vi "Force2Voltage_Linearizer_v0.vi"(6 "Z_offset [mm]":fxp<+/-,26,3>=0.02499997615814209, 7 "Scale Factor":fxp<+,10,10>=619.0, 8 "Z [mm]":fxp<+/-,26,3>, 9 "F_B [N]":fxp<+/-,25,3>, 10 "F_G [N]":fxp<+/-,25,3>, 11 "F_R [N]":fxp<+/-,25,3>) -> (1 "V_B [V]":fxp<+/-,20,5>, 2 "V_G [V]":fxp<+/-,20,5>, 3 "V_R [V]":fxp<+/-,20,5>)   [LabVIEW 2020, in "FPGA functions.lvlib"]
doc: "Linearizing actuation force to electrode voltages. \n\nThis implements the feedback linearization block!"
uses:
  FPGA functions.lvlib
  <vilib>/Platform/TimedLoop/XDataNode/timing_clust.ctl
  <vilib>/Platform/TimedLoop/XDataNode/nitl_modes.ctl
  <vilib>/Platform/TimedLoop/XDataNode/wakeup.ctl
  <vilib>/rvi/FXPMathLib/FxpSqrt/subVIs/nifxpmath_Sqrt_SimConfig.ctl
  <vilib>/fxp/LVFixedPointOverflowPolicyTypeDef.ctl
  <vilib>/rvi/Emulation/niFpgaSctlEmulationGetInTimedLoop.vi
  <vilib>/rvi/Emulation/niFpgaEmulationReportErrorSimple.vi
  <vilib>/rvi/Emulation/niFpgaGetClockAttributes.vi
  <vilib>/rvi/Emulation/niFpgaCriticalErrorInLSC.vi
  <vilib>/rvi/FXPMathLib/FxpSqrt/simVIs/DllSqrtTemp_sub.vi
  <vilib>/Platform/TimedLoop/XDataNode/XDataNode.xnode
  <vilib>/rvi/FXPMathLib/FxpSqrt/XNode/nifxpmath_Sqrt.xnode
  <vilib>/rvi/FXPMathLib/FxpAdd/XNode/nifxpmath_Add.xnode
  <vilib>/rvi/FXPMathLib/FxpMul/XNode/nifxpmath_Multiplier.xnode
  <vilib>/Platform/TimedLoop/XDataNode/XDNodeRunTimeDep.lvlib
  <vilib>/rvi/FXPMathLib/sim/FxpSim.dll
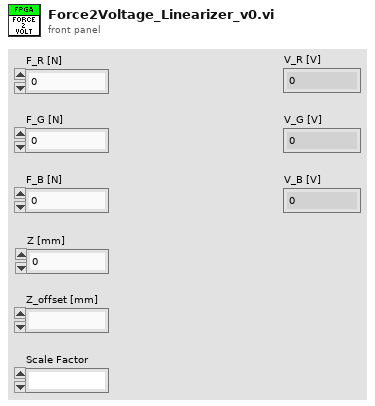
[diagram p1: front panel]
types:
  T1 = typedef "XDNodeRunTimeDep.lvlib/timing_clust.ctl" = cluster{"Expected End [f-1]":u64, "Actual End [f-1]":u64, "Finished Late? [f-1]":bool, "Expected End [i-1]":u64, "Actual End [i-1]":u64, "Finished Late? [i-1]":bool, "Expected Start [i]":u64, "Actual Start [i]":u64, "Expected Start [f]":u64, "Actual Start [f]":u64, "Source Name":string, "Structure Name":string, "Period":i64, "Deadline":i64, "Offset":i64, "Start":i64, "Priority":i32, "Timeout":i32, "Mode":T2, "Wakeup Reason":T3, "Error":errorcluster, "Source Type":string, "Secondary Source Type":string, "Global End Time":u64, "Global Start Time":u64, "Frame Duration":u64, "Iteration Duration":u64, "Assigned CPU":i32, "I/O Scan Engine Mode":u32}
  T2 = typedef "XDNodeRunTimeDep.lvlib/nitl_modes.ctl" = enum32{"No Change", "Process missed periods, maintain original phase", "Discard missed periods, maintain original phase", "Process missed periods, ignore original phase", "Discard missed periods, ignore original phase"}
  T3 = typedef "XDNodeRunTimeDep.lvlib/wakeup.ctl" = enum32{"Normal", "Aborted", "Asynchronous wakeup", "Timing source error", "Timed loop error", "Timeout"}
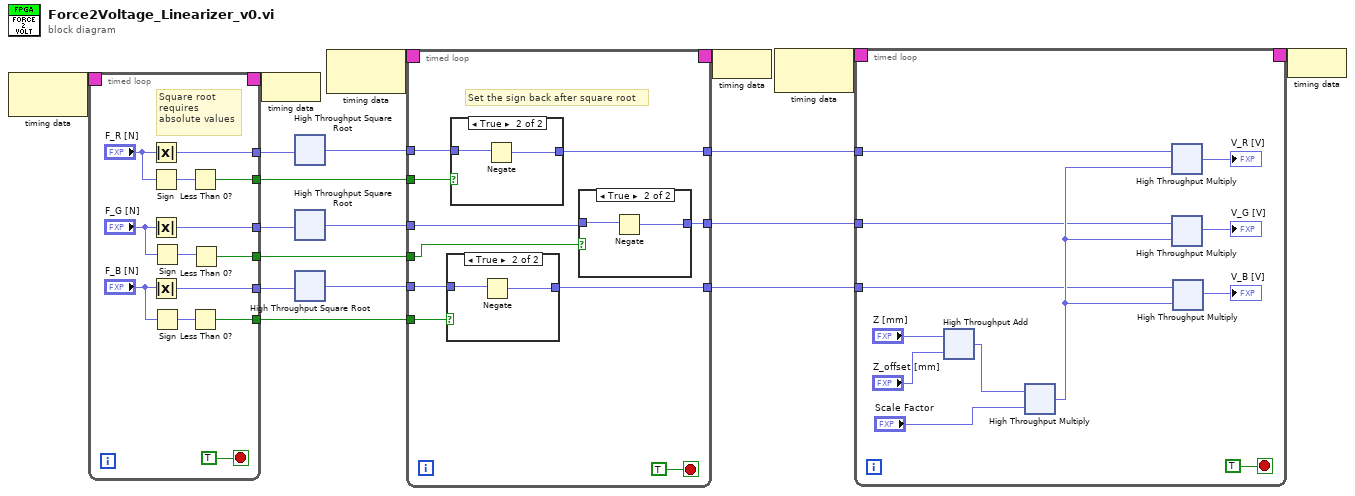
[diagram p0: block diagram]
diagram:
  n1 = node-c288() -> (w13:T1)  [unwired: 1 in]
  n2 = timed-loop {
    timing: w13 -> [_]
    timing-out: [_] -> w12
    tunnel: [w30] -> w18
    tunnel: [w29] -> w17
    tunnel: [w28] -> w16
    tunnel: [w23] -> w9
    tunnel: [w21] -> w6
    tunnel: [w19] -> w2
    stop <- TRUE stop-if-true
    # "Square root \nrequires \nabsolute values"
    n3 = Absolute Value(x="F_R [N]") -> (abs(x)=w30:fxp<+,25,3>)
    n4 = Sign(1:"F_R [N]") -> (0:w20:fxp<+/-,2,2>)
    n5 = Absolute Value(x="F_G [N]") -> (abs(x)=w29:fxp<+,25,3>)
    n6 = Absolute Value(x="F_B [N]") -> (abs(x)=w28:fxp<+,25,3>)
    n7 = Sign(1:"F_G [N]") -> (0:w22:fxp<+/-,2,2>)
    n8 = Sign(1:"F_B [N]") -> (0:w24:fxp<+/-,2,2>)
    n9 = Less Than 0?(x=w20) -> (x < 0?=w19:bool)
    n10 = Less Than 0?(x=w24) -> (x < 0?=w23:bool)
    n11 = Less Than 0?(x=w22) -> (x < 0?=w21:bool)
  }
  n12 = node-c288(w12) -> ()
  n13 = xnode "High Throughput Square Root"("x"=w18) -> ("sqrt(x)"=w3:fxp<+,13,2>)
  n14 = xnode "High Throughput Square Root"("x"=w17) -> ("sqrt(x)"=w5:fxp<+,13,2>)
  n15 = xnode "High Throughput Square Root"("x"=w16) -> ("sqrt(x)"=w8:fxp<+,13,2>)
  n16 = node-c288() -> (w11:T1)  [unwired: 1 in]
  n17 = timed-loop {
    timing: w11 -> [_]
    timing-out: [_] -> w10
    tunnel: w9 -> [w43]
    tunnel: w8 -> [w42]
    tunnel: [w41] -> w7
    tunnel: w6 -> [w40]
    tunnel: w5 -> [w39]
    tunnel: [w38] -> w4
    tunnel: w3 -> [w36]
    tunnel: w2 -> [w35]
    tunnel: [w34] -> w1
    stop <- TRUE stop-if-true
    # "Set the sign back after square root"
    n18 = case shown="True" w43 {
      tunnel: w42 -> [w50 w52]
      tunnel: [w50 w51] -> w41
      frame False {
      }
      frame True {
        n19 = Negate(x=w52) -> (-x=w51:fxp<+/-,14,3>)
      }
    }
    n20 = case shown="True" w35 {
      tunnel: w36 -> [w44 w46]
      tunnel: [w44 w45] -> w34
      frame False {
      }
      frame True {
        n21 = Negate(x=w46) -> (-x=w45:fxp<+/-,14,3>)
      }
    }
    n22 = case shown="True" w40 {
      tunnel: w39 -> [w47 w49]
      tunnel: [w47 w48] -> w38
      frame False {
      }
      frame True {
        n23 = Negate(x=w49) -> (-x=w48:fxp<+/-,14,3>)
      }
    }
  }
  n24 = node-c288(w10) -> ()
  n25 = node-c288() -> (w15:T1)  [unwired: 1 in]
  n26 = timed-loop {
    timing: w15 -> [_]
    timing-out: [_] -> w14
    tunnel: w7 -> [w57]
    tunnel: w4 -> [w56]
    tunnel: w1 -> [w55]
    stop <- TRUE stop-if-true
    n27 = xnode ("High Throughput Add")("x"="Z [mm]", "y"="Z_offset [mm]") -> ("x+y"=w65:fxp<+/-,27,4>)
    n28 = xnode ("High Throughput Multiply")("x"=w65, "y"="Scale Factor") -> ("x*y"=w61:fxp<+/-,37,14>)
    n29 = xnode ("High Throughput Multiply")("x"=w55, "y"=w61) -> ("x*y"=→"V_R [V]":fxp<+/-,20,5>)
    n30 = xnode ("High Throughput Multiply")("x"=w56, "y"=w61) -> ("x*y"=→"V_G [V]":fxp<+/-,20,5>)
    n31 = xnode ("High Throughput Multiply")("x"=w57, "y"=w61) -> ("x*y"=→"V_B [V]":fxp<+/-,20,5>)
  }
  n32 = node-c288(w14) -> ()
